vi "CANFrame2.0_Avg_Length.vi"(0 "Payload Size (bytes)":i32, 1 "Extended ID?":bool) -> (5 "Avg.Length (bits)":i32)   [LabVIEW 2019, in "XNET-Bus-Load-Calculator.lvlib" / "CANBus_Load_Calculator.lvclass"]
uses:
  CANBus_Load_Calculator.lvclass
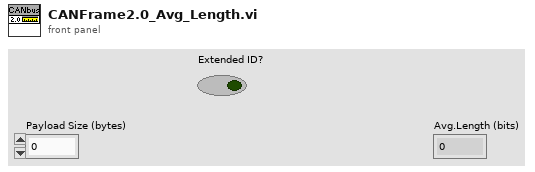
[diagram p1: front panel]
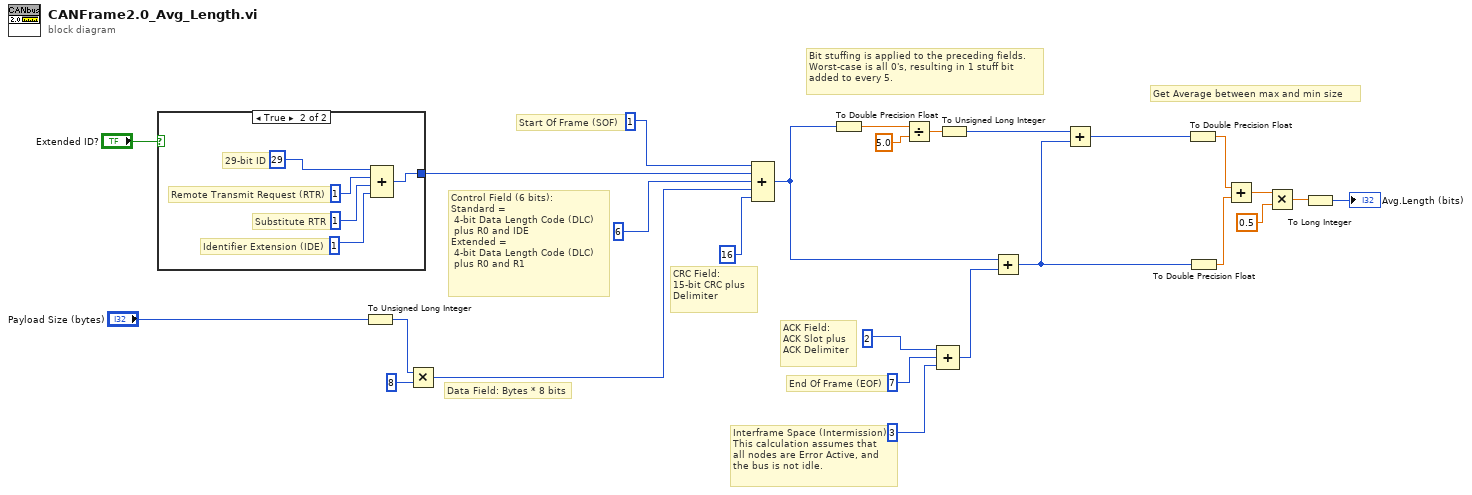
[diagram p0: block diagram]
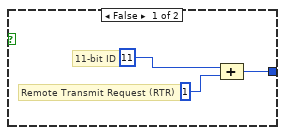
[diagram p2: hidden frame]
diagram:
  # "Get Average between max and min size"
  # "Interframe Space (Intermission)\nThis calculation assumes that\nall nodes are Error Active, and\nthe bus is not idle."
  # "End Of Frame (EOF)"
  # "ACK Field:\nACK Slot plus\nACK Delimiter"
  # "Bit stuffing is applied to the preceding fields.\nWorst-case is all 0's, resulting in 1 stuff bit\nadded to every 5."
  # "CRC Field:\n15-bit CRC plus \nDelimiter"
  # "Data Field: Bytes * 8 bits"
  # "Control Field (6 bits):\nStandard = \n 4-bit Data Length Code (DLC)\n plus R0 and IDE\nExtended = \n 4-bit Data Length Code (DLC)\n plus R0 and R1"
  # "Start Of Frame (SOF)"
  n1 = case shown="True" "Extended ID?" {
    tunnel: [w27 w32] -> w2
    frame False {
      # "Remote Transmit Request (RTR)"
      # "11-bit ID"
      n2 = Compound Arithmetic op=unknown(u32 11, u32 1) -> (w27:u32)
    }
    frame True {
      # "Identifier Extension (IDE)"
      # "Substitute RTR"
      # "Remote Transmit Request (RTR)"
      # "29-bit ID"
      n3 = Compound Arithmetic op=unknown(u32 29, u32 1, u32 1, u32 1) -> (w32:u32)
    }
  }
  n4 = To Unsigned Long Integer(number="Payload Size (bytes)") -> (unsigned 32bit integer=w12:u32)
  n5 = Multiply(x=w12, y=u32 8) -> (x*y=w23:u32)
  n6 = Compound Arithmetic op=ADD(u32 1, w2, u32 6, w23, u32 16) -> (w18:u32)
  n7 = To Double Precision Float(number=w18) -> (double precision float=w11:dbl)
  n8 = Divide(x=w11, y=5.0) -> (x/y=w16:dbl)
  n9 = Compound Arithmetic op=unknown(u32 2, u32 7, u32 3) -> (w17:u32)
  n10 = To Unsigned Long Integer(number=w16) -> (unsigned 32bit integer=w15:u32)
  n11 = Add(x=w18, y=w17) -> (x+y=w9:u32)
  n12 = Add(x=w15, y=w9) -> (x+y=w10:u32)
  n13 = To Double Precision Float(number=w10) -> (double precision float=w8:dbl)
  n14 = To Double Precision Float(number=w9) -> (double precision float=w7:dbl)
  n15 = Add(x=w8, y=w7) -> (x+y=w6:dbl)
  n16 = Multiply(x=w6, y=0.5) -> (x*y=w4:dbl)
  n17 = To Long Integer(number=w4) -> (32bit integer=→"Avg.Length (bits)":i32)
